vi "Configure.vi"(8 "error in (no error)":errorcluster caption="错误输入（无错误）", 11 "Simulation Source 输入":refnum<class "Simulation Source.lvclass">) -> (0 "error out":errorcluster caption="错误输出", 3 "Simulation Source 输出":refnum<class "Simulation Source.lvclass">)   [LabVIEW 2020, in "Simulation Source.lvlib" / "Simulation Source.lvclass"]
uses:
  Simulation Source.lvclass
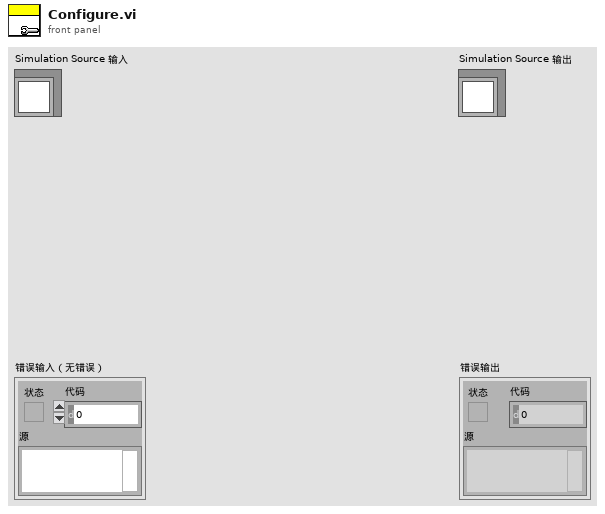
[diagram p1: front panel]
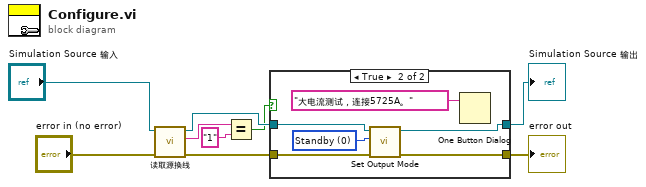
[diagram p0: block diagram]
diagram:
  n1 = call "读取源换线.vi"("error in (no error)"="error in (no error)", "多功能校准源接口输入"="Simulation Source 输入") -> ("error out"=w9:errorcluster, "源换线"=w6:string, "多功能校准源接口输出"=w8:refnum<class "Simulation Source.lvclass">)  [unwired: 7 in]
  n2 = Equal?(x=w6, y="1") -> (x = y?=w7:bool)
  n3 = case shown="True" w7 {
    tunnel: w8 -> [w11 w17]
    tunnel: [w11 w14] -> w3
    tunnel: w9 -> [w10 w13]
    tunnel: [w10 w12] -> w1
    frame False {
    }
    frame True {
      w16 = u32 0 items=["Standby", "Operate"] ("Output Mode")
      n4 = call-dynamic "Set Output Mode.vi"("error in (no error)"=w13, "Output Mode"=w16, "Simulation Source 输入"=w17) -> ("error out"=w12:errorcluster, "Simulation Source 输出"=w14:refnum<class "Simulation Source.lvclass">)  [unwired: 7 in]
      n5 = One Button Dialog(message="大电流测试，连接5725A。" ("消息")) -> ()  [unwired: 1 in, 1 out]
    }
  }
  "error out" <- w1
  "Simulation Source 输出" <- w3
